vi "AutoClimbNavX.vi"(8 "Stage":i8, 9 "Elevator Encoder":i32, 10 "Horse Encoder":i32) -> (1 "Elevator Output":dbl, 2 "Horse Output":dbl)   [LabVIEW 2018]
uses:
  <vilib>/addons/control/pid/pid.llb/PID (DBL).vi
  <vilib>/addons/control/pid/NI_PID_pid.lvlib
panel:
  in  "Elevator PID Gains":T1={"proportional gain (Kc)"=1e-06, "integral time (Ti, min)"=0.0, "derivative time (Td, min)"=0.0}
  in  "Horse PID Gains":T1={"proportional gain (Kc)"=1e-05, "integral time (Ti, min)"=0.0, "derivative time (Td, min)"=0.0}
  in  "Elevator Setpoint":i32
  in  "Horse Setpoint":i32=-180000
  in  "Elevator Gyro P Val":dbl=10.0
  in  "Horse Gyro P Val":dbl=-10.0
  out "Gyro Values":T2
  # "Horse: Neg P gyro val\nElevator: Pos gyro val\n\nHorse: Pos gain\nElevator: Pos gain"
  # "Neg"
  # "Pos"
  # "Horse drive P control negated for Alpha"
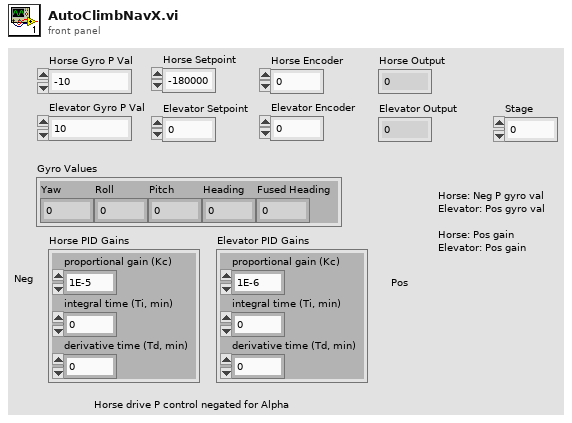
[diagram p1: front panel]
types:
  T1 = cluster{"proportional gain (Kc)":dbl, "integral time (Ti, min)":dbl, "derivative time (Td, min)":dbl}
  T2 = cluster{"Yaw":dbl, "Roll":dbl, "Pitch":dbl, "Heading":dbl, "Fused Heading":dbl}
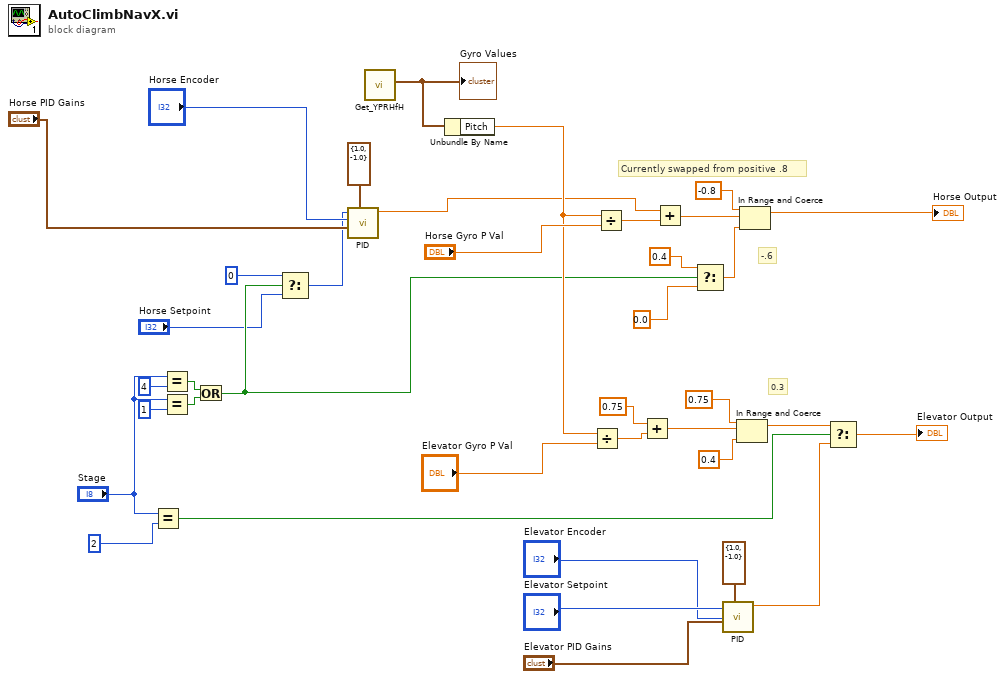
[diagram p0: block diagram]
diagram:
  # "Currently swapped from positive .8"
  # "0.3"
  # "-.6"
  n1 = Equal?(x="Stage", y=i8 2) -> (x = y?=w14:bool)
  n2 = Equal?(x="Stage", y=i8 4) -> (x = y?=w12:bool)
  n3 = Equal?(x="Stage", y=i8 1) -> (x = y?=w11:bool)
  n4 = Or(x=w12, y=w11) -> (x .or. y?=w3:bool)
  n5 = Select(t=i8 0 ("y"), s=w3, f="Horse Setpoint") -> (s? t:f=w1:i32)
  n6 = call-poly <vilib>:"PID.vi"("output range"=cluster{"output high":dbl, "output low":dbl} {"output high"=1.0, "output low"=-1.0}, "PID gains"="Horse PID Gains", "process variable"="Horse Encoder", "setpoint"=w1) -> ("output"=w25:dbl)  [unwired: 6 in, 1 out]
  n7 = call <vilib>:"Get_YPRHfH.vi"() -> ("YRPHfH"=w38:T2)  [unwired: 11 in]
  "Gyro Values" <- w38
  n8 = Unbundle By Name(w38) -> ("Pitch"=w31:dbl)
  n9 = Divide(x=w31, y="Elevator Gyro P Val") -> (x/y=w28:dbl)
  n10 = Divide(x=w31, y="Horse Gyro P Val") -> (x/y=w29:dbl)
  n11 = Add(x=0.75, y=w28) -> (x+y=w27:dbl)
  n12 = Add(x=w25, y=w29) -> (x+y=w30:dbl)
  n13 = Select(t=0.4, s=w3, f=0.0 ("lower limit")) -> (s? t:f=w6:dbl)
  n14 = call-poly <vilib>:"PID.vi"("output range"=cluster{"output high":dbl, "output low":dbl} {"output high"=1.0, "output low"=-1.0}, "PID gains"="Elevator PID Gains", "process variable"="Elevator Encoder", "setpoint"="Elevator Setpoint") -> ("output"=w17:dbl)  [unwired: 6 in, 1 out]
  n15 = In Range and Coerce(upper limit=0.75, x=w27, lower limit=0.4) -> (coerced(x)=w16:dbl)  [unwired: 1 out]
  n16 = In Range and Coerce(upper limit=-0.8, x=w30, lower limit=w6) -> (coerced(x)=→"Horse Output":dbl)  [unwired: 1 out]
  n17 = Select(t=w16, s=w14, f=w17) -> (s? t:f=→"Elevator Output":dbl)
